vi "RoboDisplay7beingedited.vi"() -> ()   [LabVIEW 2015]
uses:
  GlobalDisplayIndex.vi
  GlobalDataSize.vi
  GlobalInitialParamVals.vi
  GlobalErrorCAN_ID.vi
  ErrorPrevValues.vi
  GlobalErrorCluster.vi
  GlobalLabVIEWStart.vi
  GlobalSpeedUpdateTime.vi
  GlobalPlotUpdateTime.vi
  GlobalSpeedArray.vi
  GlobalDataSelectArray.vi
  GlobalFavoritesList.vi
  GlobalFavorites.vi
  GlobalParamSize.vi
  GlobalFavoriteNames.vi
  GlobalDataFileRefnum7.vi
  GlobalDataPath7.vi
  GlobalRobotOffCheck.vi
  GlobalPrevPage.vi
  GlobalErrorIndex.vi
  GlobalBatteryVoltageID.vi
  GlobalLoadedParams.vi
panel:
  in  "?":T1
  in  "Select":T1
  in  "Select 4":T1
  in  "Select 3":T1
  in  "Load param display file":bool
  out "MCU Elapsed mS 2":u32
  in  "Collect Data":bool
  out "Boolean":bool
  out "graph2labels":string[](array[string])
  out "graph1labels":string[](array[string])
  out "BATTERY VOLTAGE":dbl(knob) scale=20.0..30.0 scale format="%#_3g"
  in  "Tab Control":T2(tab)=enum."Display Data"
  out "Fav Error":bool[](array[boolean])
  in  "Remove":T3
  in  "Fav":T1
  in  "Commit":T4
  out "WAIT":bool
  in  "Reset default":bool
  out "Param #":dbl[](array[numeric])
  in  "Select 2":T5
  in  "Fav Input":dbl[](array[numeric])
  out "Value":dbl[](array[numeric])
  in  "Load":bool
  in  "Save":bool
  out "error":bool[](array[boolean])
  out "Param value":dbl[](array[numeric])
  out "Param #":dbl[](array[numeric])
  out "Param Name":string[](array[string])
  in  "Input":dbl[](array[numeric])
  in  "Page Select":dbl min=0.0 max=50.0 step=1.0
  out "Favorite Parameters":string[](array[string])
  in  "save data":bool
  in  "load data":bool
  out "Value 2":dbl[](array[numeric])
  out "Value 1":dbl[](array[numeric])
  out "Data # 2":dbl[](array[numeric])
  out "Data #":dbl[](array[numeric])
  out "Indicator":bool[](array[boolean])
  out "Array":string[](array[string])
  in  "Page":dbl min=0.0 max=50.0 step=1.0
  out "Number\nSelected":dbl
  out "Indicator 2":bool[](array[boolean])
  out "Array 2":string[](array[string])
  out "Results":T6(array[cluster])
  in  "Search":string
  in  "Search \nButton":bool
  out "# of Results":i32
  in  "Speed Sel 2":enum32{"Slow", "Medium", "Fast"}[](array[radio])
  out "Speed 3":u32[](array[colorbox])
  out "Data Names 2":string[](array[string])
  out "Channel # 2":i16[](array[numeric])
  out "Data Value 2":sgl[](array[numeric]) format="%#_4g"
  out "Speed 2":u32[](array[colorbox])
  out "Data Names 1":string[](array[string])
  out "Channel # 1":i16[](array[numeric])
  out "Data Value 1":sgl[](array[numeric]) format="%#_4g"
  in  "One1":bool[](array[boolean])
  in  "One2":bool[](array[boolean])
  in  "Two1":bool[](array[boolean])
  in  "Two2":bool[](array[boolean])
  in  "Speed Sel":enum32{"Slow", "Medium", "Fast"}[](array[radio])
  in  "Clear Errors":bool
  in  "Pause Button":bool
  out "Error Description":string[](array[string])
  out "Board":string[](array[string])
  out "Error Name":string[](array[string])
  out "Freq.":dbl[](array[numeric])
  out "Time":dbl[](array[numeric])
  out "error message":bool
  out "Board Name 1":string
  out "Graph One":cluster{"Array":u32[], "Array 2":sgl[]}[](graph)
  in  "Graph\non":bool
  out "Error Name 1":string
  out "MCU Elapsed mS":u32 format="%<%H:%M:%S>t"
  in  "stop":bool
  out "Graph Two":cluster{"Array":u32[], "Array 2":sgl[]}[](graph)
  # "Robot Time:"
  # "ms timer:"
  # "DATA COLLECTION"
  # "Board"
  # "OFF"
  # "ON"
  # "Error Name"
  # "RoboDAQ\n\n(Version 7)\n\n\n\n\n\n\nCreated by: John Buzzi, Jason Cortell, Katie Hartl, Carlos Arango\n\nFall 2009"
  # "PLEASE LOOK AT SUGGESTIONS\nTAB IF YOU HAVE HELPFUL \nCOMMENTS!!"
  # "Favorites"
  # "Press [Home] to increment\nPress [End] to decrement"
  # "Press [Page Up] to increment\nPress [Page Down] to decrement"
  # "Select"
  # "Select"
  # "MAX ALLOWED: 48"
  # "NOT WORKING YET\n.\n.\n.\n.\n.\n.\n.\n......................."
  # "CAN ID"
  # "Name"
  # "Search Field"
  # "Note: Add function does not work yet"
  # "# of hits"
  # "Graphs"
  # "Graphs"
  # "Speed\n(S)   (M)   (F)"
  # "Speed\n(S)   (M)   (F)"
  # "Speed"
  # "Speed"
  # "Channel Name"
  # "One"
  # "Two"
  # "Channel Name"
  # "One"
  # "Two"
  # "SUGGESTIONS (double click text box to edit)\n\nMy to do list:\nFix error handling so that it works in the more advanced way that I had intended\nFix bug with speed select when data is de-selected and speeds are incorrect\nradio buttons\nload save data\nadd data by number\nmake index bigger\nslow default speed\n\n\nOther Suggestions/Comments (please add user input so that I can make the program better)\n- (nac) Change default folder for can_id.h and error_id.h to the Ranger Configuration folder\n\n\n\n\nNote: Strikeout = fixed"
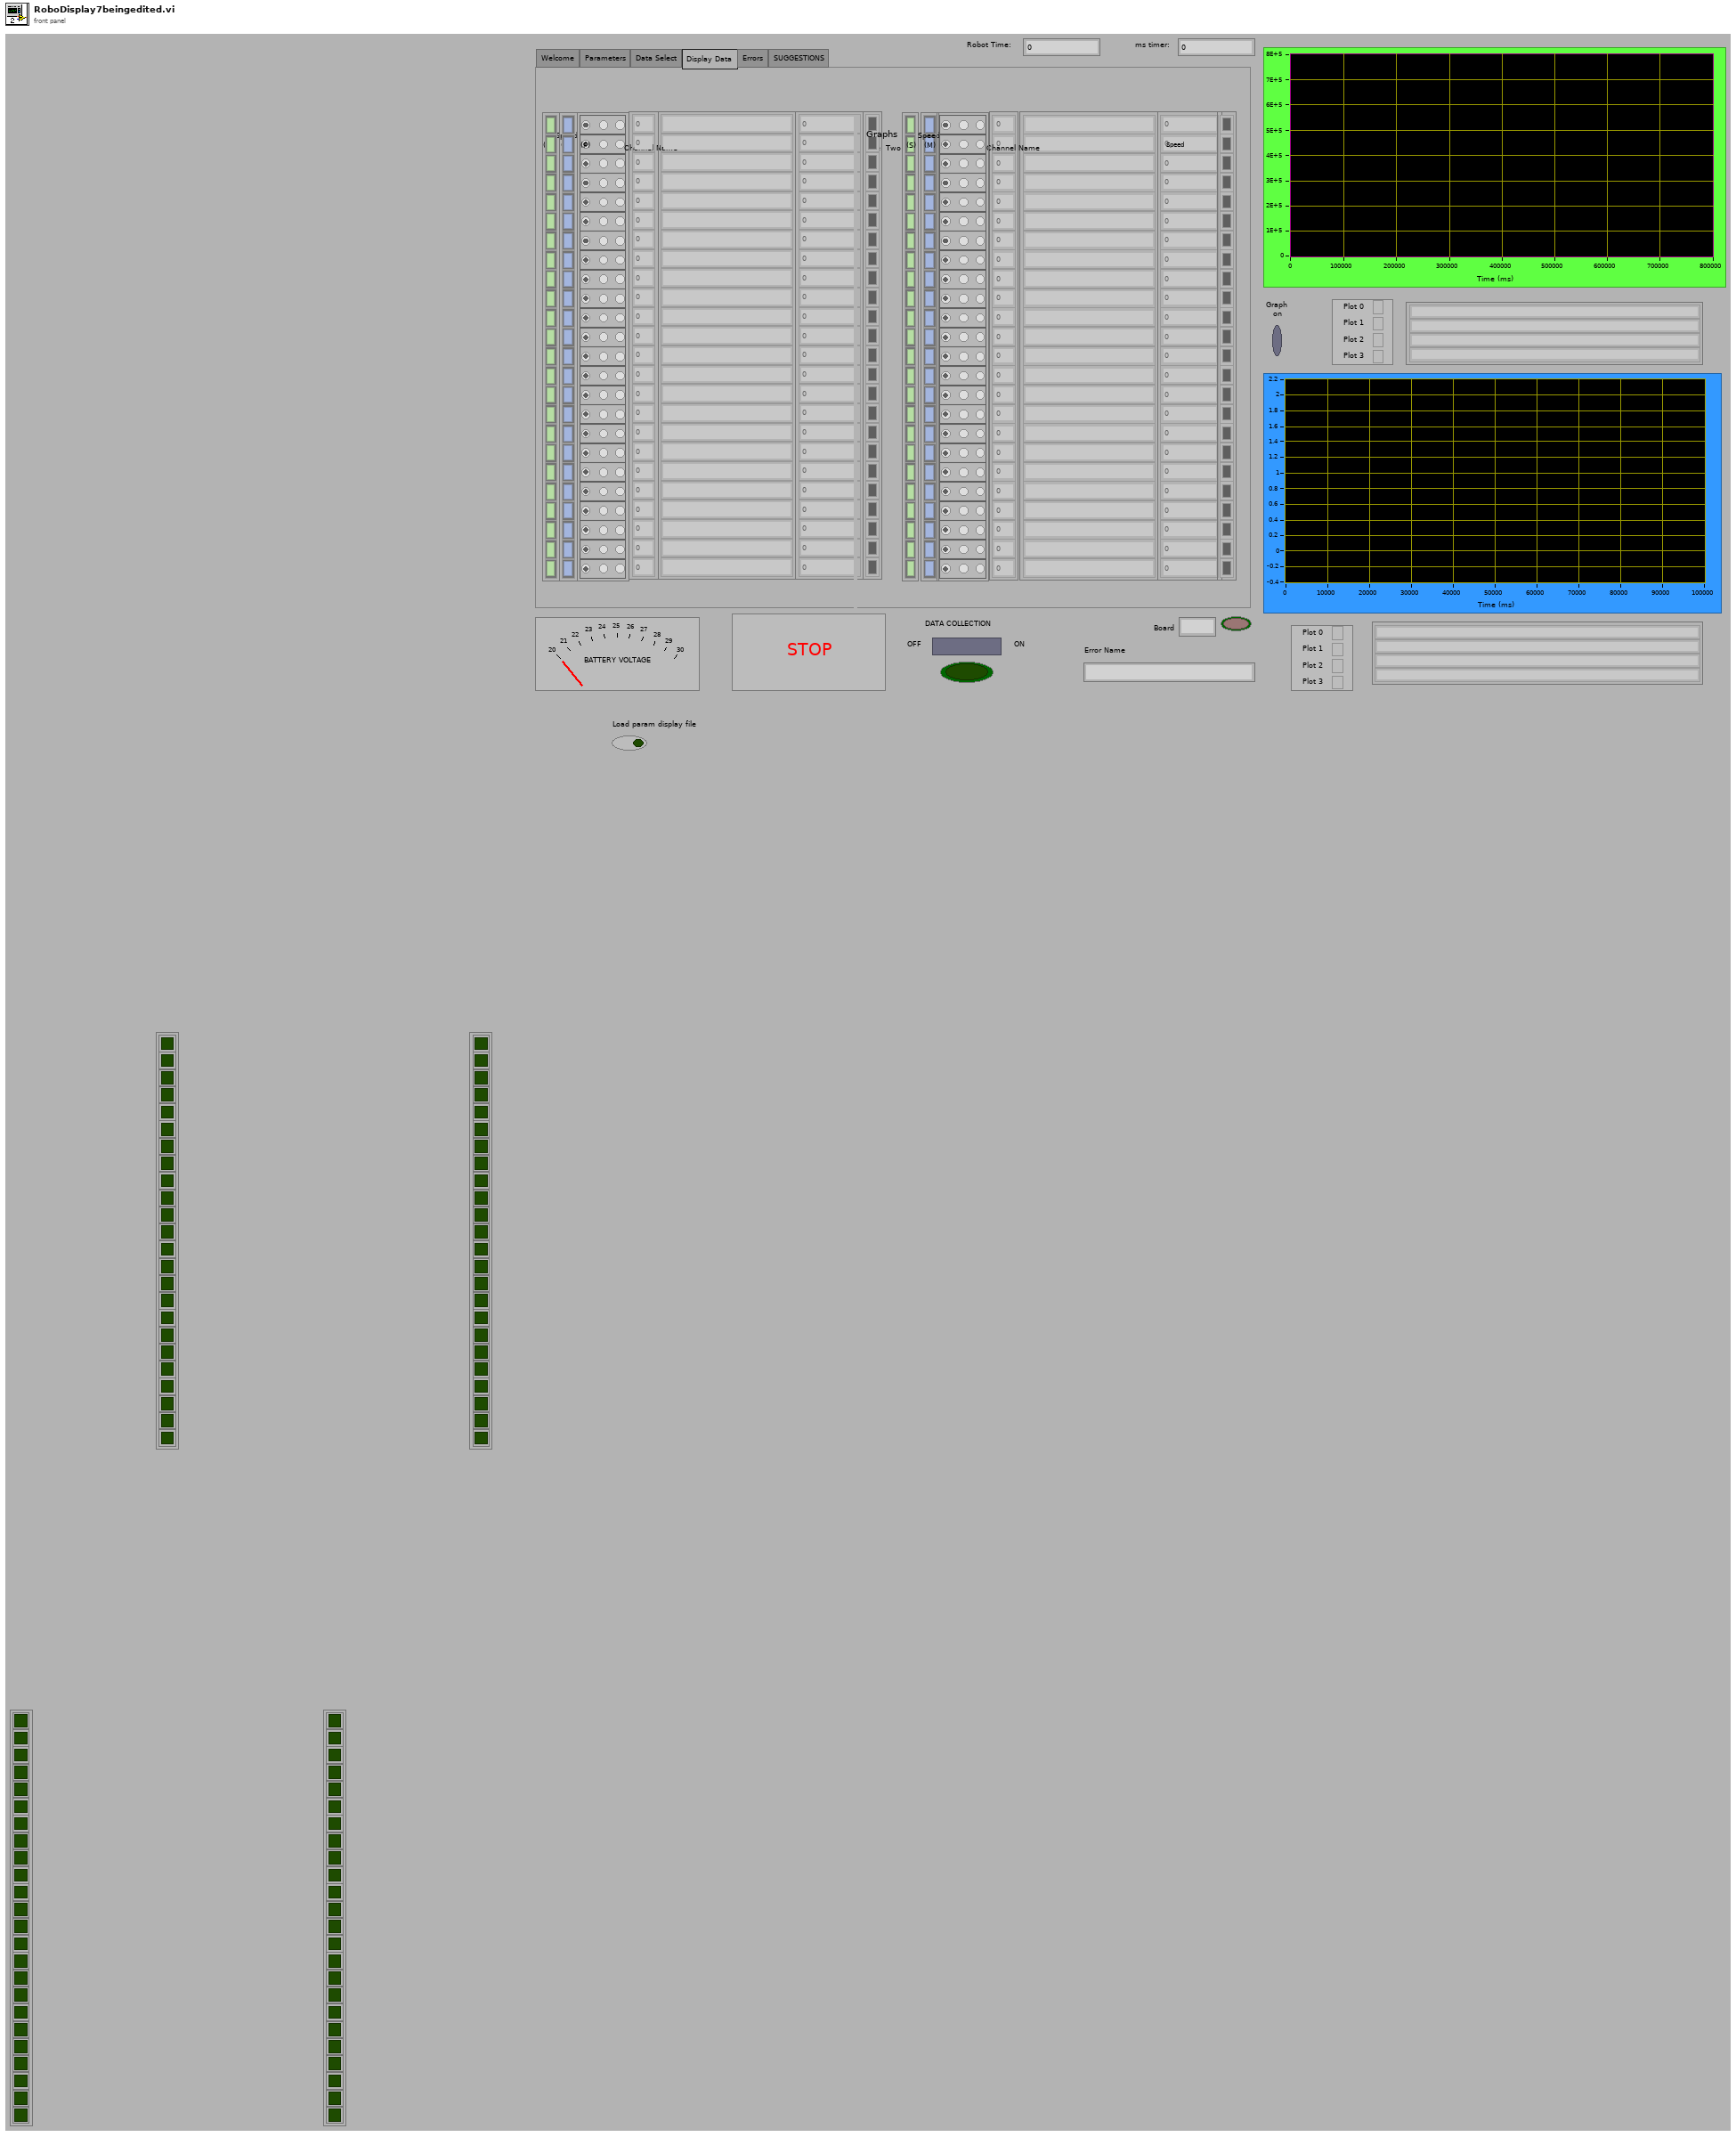
[diagram p1: front panel]
types:
  T1 = cluster{"Boolean 2":bool, "Boolean 3":bool, "Boolean 4":bool, "Boolean 5":bool, "Boolean 6":bool, "Boolean 7":bool, "Boolean 8":bool, "Boolean 9":bool, "Boolean 10":bool, "Boolean 11":bool, "Boolean 12":bool, "Boolean 13":bool, "Boolean 14":bool, "Boolean 15":bool, "Boolean 16":bool, "Boolean 17":bool, "Boolean 18":bool, "Boolean 19":bool, "Boolean 20":bool, "Boolean 21":bool, "Boolean 22":bool, "Boolean 23":bool, "Boolean 24":bool, "Boolean 25":bool}
  T2 = enum32{"Welcome", "Parameters", "Data Select", "Display Data", "Errors", "SUGGESTIONS"}
  T3 = cluster{"X button":bool, "X button 2":bool, "X button 3":bool, "X button 4":bool, "X button 5":bool, "X button 6":bool, "X button 7":bool, "X button 8":bool, "X button 9":bool, "X button 10":bool, "X button 11":bool, "X button 12":bool, "X button 13":bool, "X button 14":bool, "X button 15":bool, "X button 16":bool, "X button 17":bool, "X button 18":bool, "X button 19":bool, "X button 20":bool}
  T4 = cluster{"Boolean":bool, "Boolean 2":bool, "Boolean 3":bool, "Boolean 4":bool, "Boolean 5":bool, "Boolean 6":bool, "Boolean 7":bool, "Boolean 8":bool, "Boolean 9":bool, "Boolean 10":bool, "Boolean 11":bool, "Boolean 12":bool, "Boolean 13":bool, "Boolean 14":bool, "Boolean 15":bool, "Boolean 16":bool, "Boolean 17":bool, "Boolean 18":bool, "Boolean 19":bool, "Boolean 20":bool}
  T5 = cluster{"Boolean":bool, "Boolean 2":bool, "Boolean 3":bool, "Boolean 4":bool, "Boolean 5":bool, "Boolean 6":bool, "Boolean 7":bool, "Boolean 8":bool, "Boolean 9":bool, "Boolean 10":bool, "Boolean 11":bool, "Boolean 12":bool, "Boolean 13":bool, "Boolean 14":bool, "Boolean 15":bool, "Boolean 16":bool, "Boolean 17":bool, "Boolean 18":bool, "Boolean 19":bool, "Boolean 20":bool, "Boolean 21":bool, "Boolean 22":bool, "Boolean 23":bool, "Boolean 24":bool}
  T6 = cluster{"Result Index":dbl, "Results 3":string, "Boolean 2":bool}[]
  T7 = cluster{"Error ID":i32, "Board ID":i32, "Time":u32, "Frequency":i32}[]
  T8 = enum16{"open", "replace", "create", "open or create", "replace or create", "replace or create with confirmation"}
  T9 = cluster{"Numeric":dbl, "String":string, "ignore case? (F)":bool}
  T10 = cluster{"Select 4[0]":bool, "Select 4[1]":bool, "Select 4[2]":bool, "Select 4[3]":bool, "Select 4[4]":bool, "Select 4[5]":bool, "Select 4[6]":bool, "Select 4[7]":bool, "Select 4[8]":bool, "Select 4[9]":bool, "Select 4[10]":bool, "Select 4[11]":bool, "Select 4[12]":bool, "Select 4[13]":bool, "Select 4[14]":bool, "Select 4[15]":bool, "Select 4[16]":bool, "Select 4[17]":bool, "Select 4[18]":bool, "Select 4[19]":bool, "Select 4[20]":bool, "Select 4[21]":bool, "Select 4[22]":bool, "Select 4[23]":bool}
  T11 = cluster{"Select 3[0]":bool, "Select 3[1]":bool, "Select 3[2]":bool, "Select 3[3]":bool, "Select 3[4]":bool, "Select 3[5]":bool, "Select 3[6]":bool, "Select 3[7]":bool, "Select 3[8]":bool, "Select 3[9]":bool, "Select 3[10]":bool, "Select 3[11]":bool, "Select 3[12]":bool, "Select 3[13]":bool, "Select 3[14]":bool, "Select 3[15]":bool, "Select 3[16]":bool, "Select 3[17]":bool, "Select 3[18]":bool, "Select 3[19]":bool, "Select 3[20]":bool, "Select 3[21]":bool, "Select 3[22]":bool, "Select 3[23]":bool}
  T12 = cluster{"Numeric":dbl, "String":string, "ignore case? (F)":bool}[]
  T13 = cluster{"Frequency":dbl, "Description":string, "Error Name":string, "Board Name":string, " Board Source":dbl, "Timestamp":dbl}[]
  T14 = cluster{"Frequency":dbl, "Description":string, "Error Name":string, "Board Name":string, " Board Source":dbl, "Timestamp":dbl}
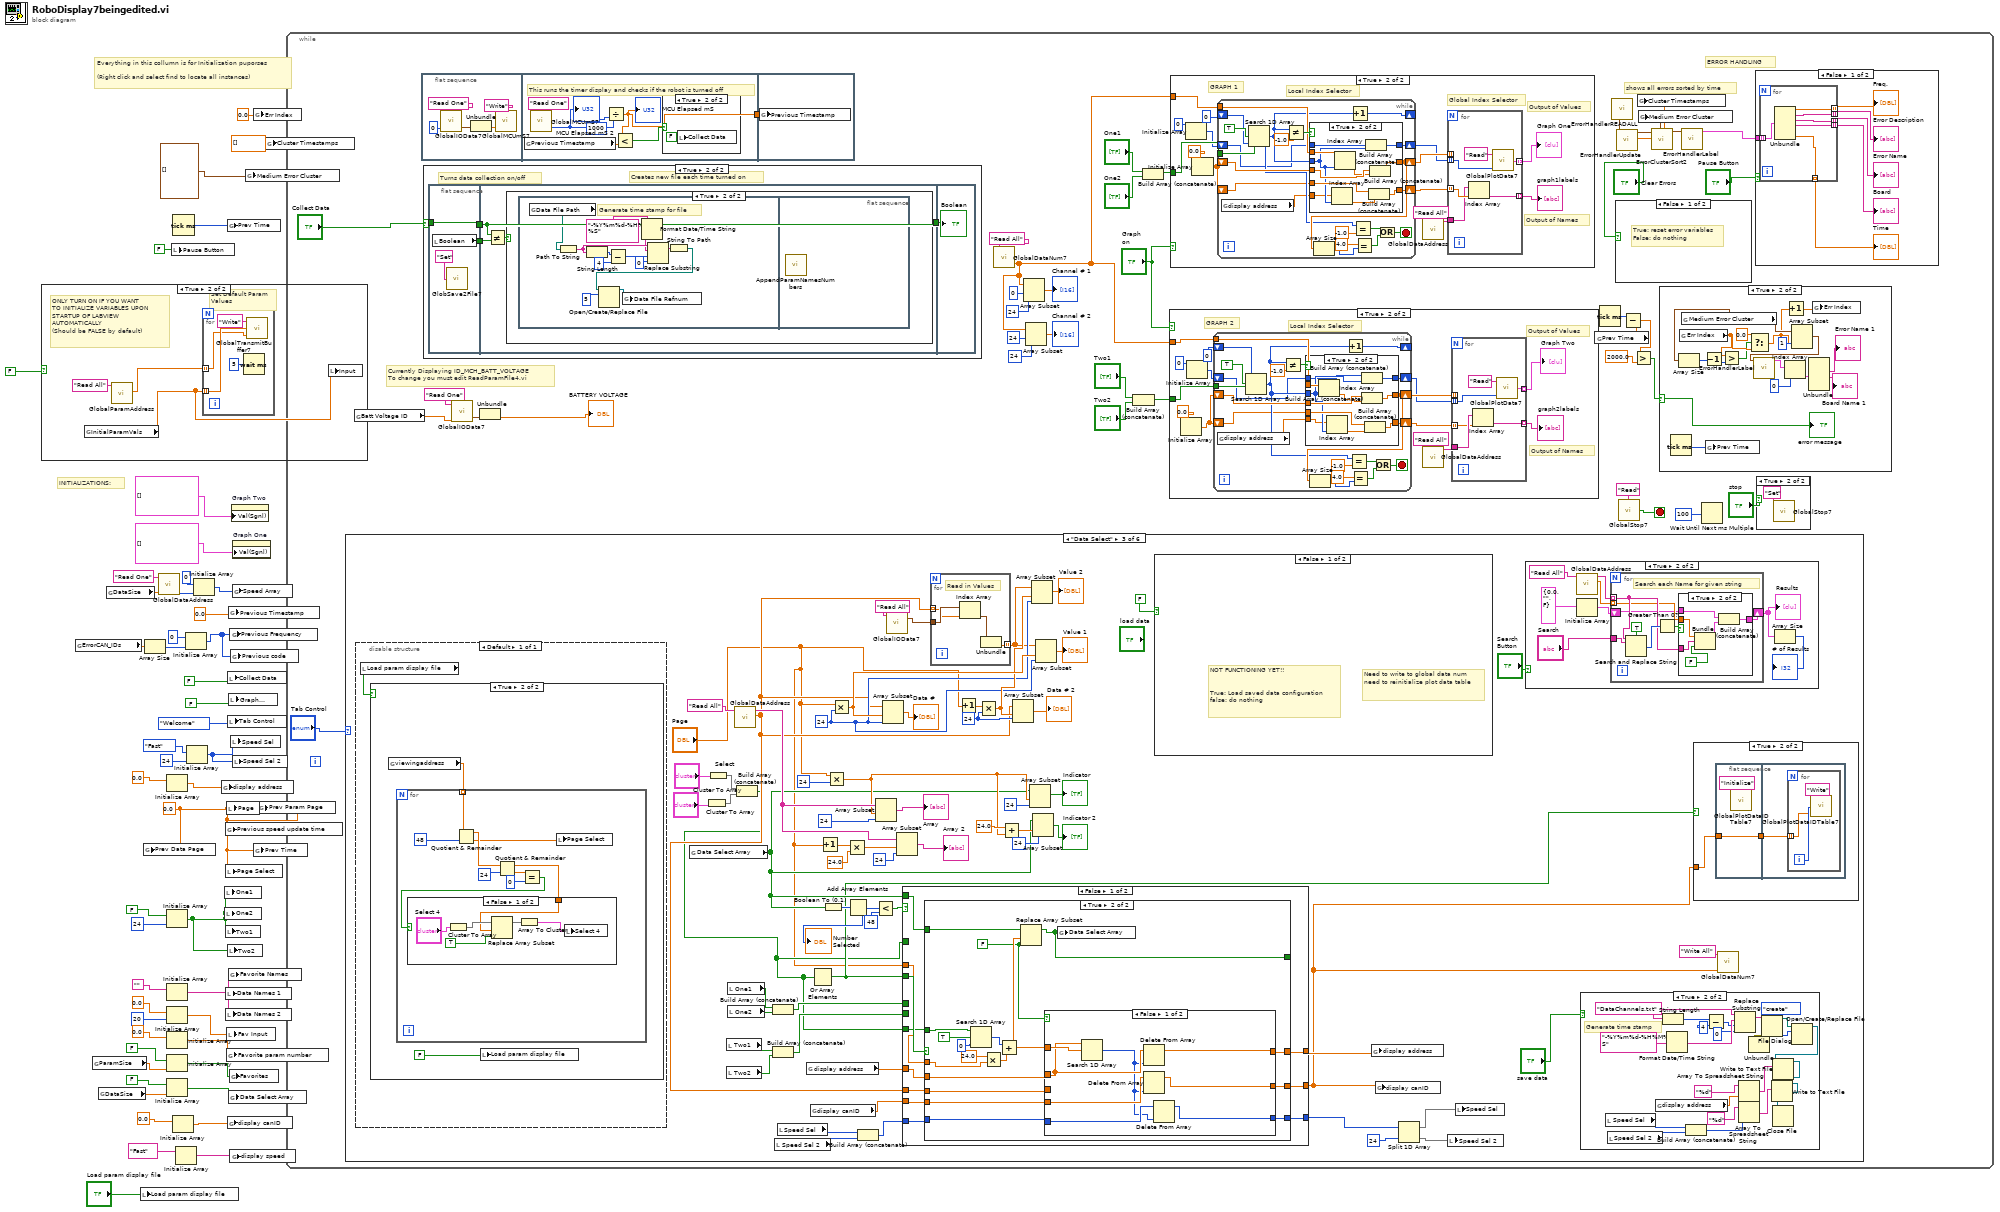
[diagram p0: block diagram]
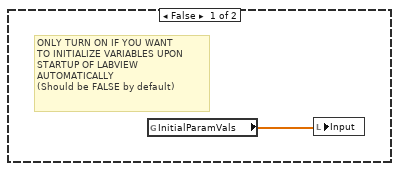
[diagram p2: hidden frame]
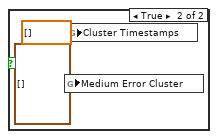
[diagram p3: hidden frame]
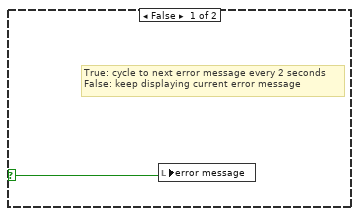
[diagram p4: hidden frame]
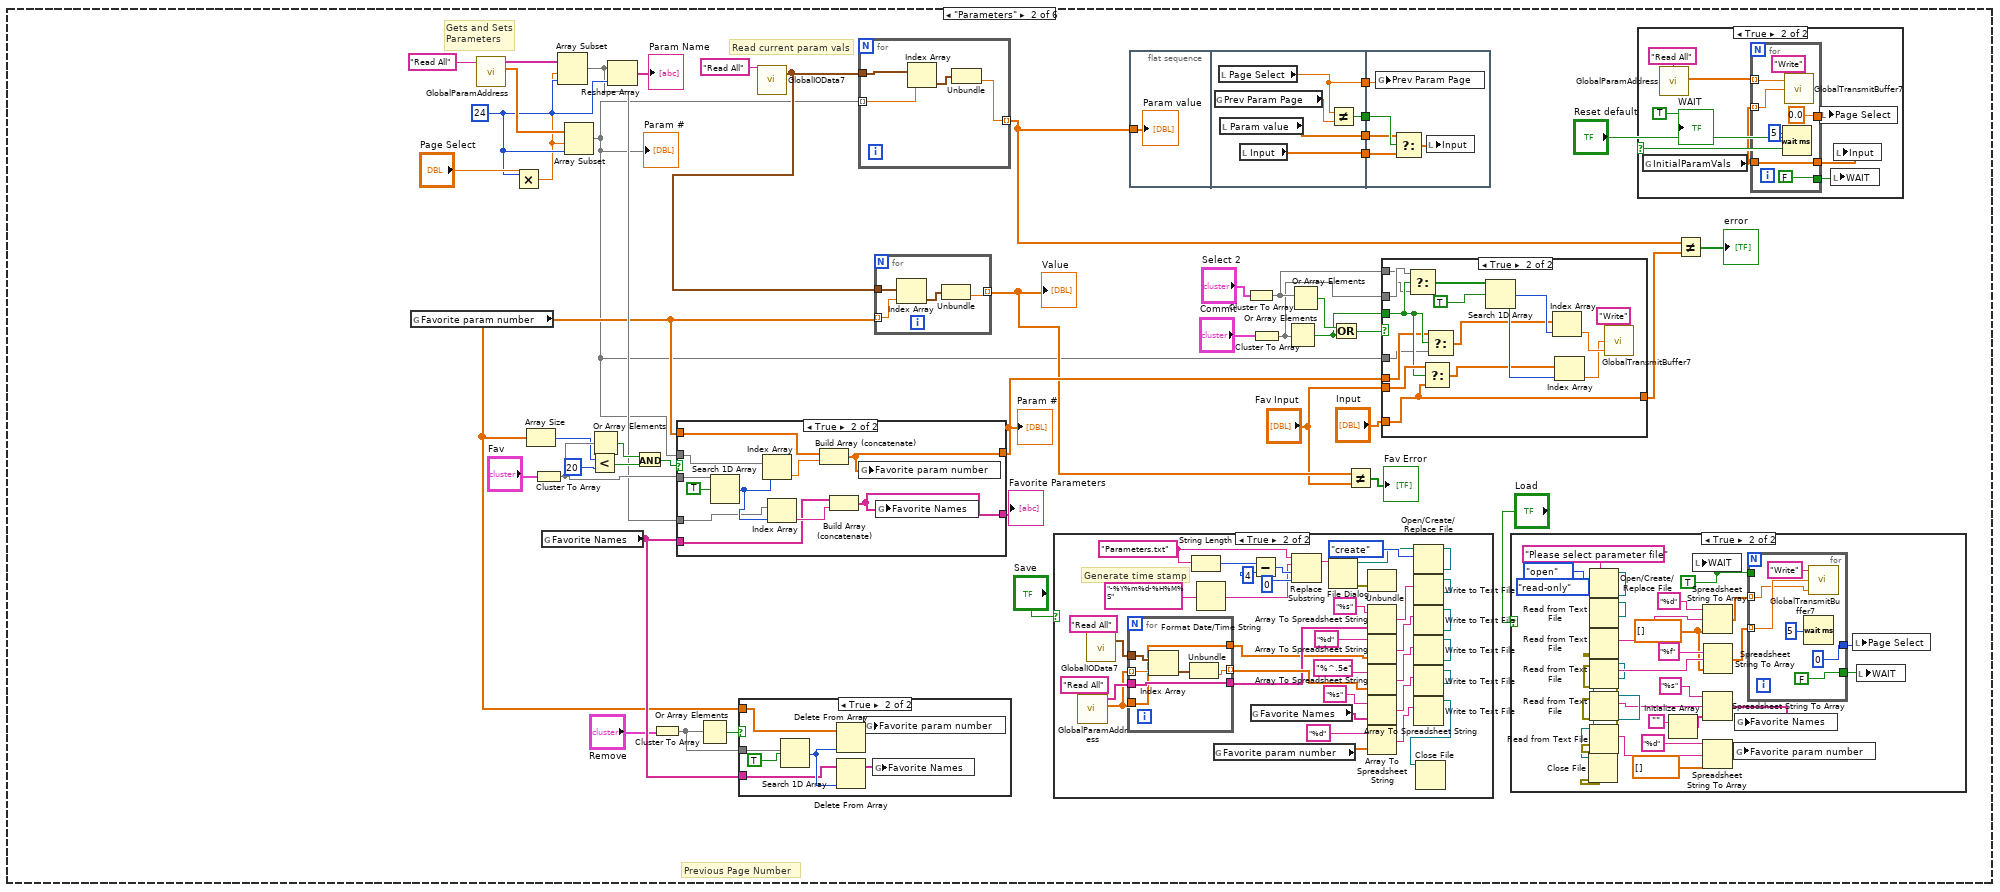
[diagram p12: hidden frame]
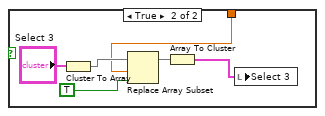
[diagram p20: hidden frame]
diagram:
  w14 = 0.0 ("Previous speed update time")
  # "Everything in this collumn is for Initialization puporses\n\n(Right click and select find to locate all instances)"
  # "INITIALIZATIONS:"
  n1 = case shown="True" FALSE {
    frame False {
      # "ONLY TURN ON IF YOU WANT\nTO INITIALIZE VARIABLES UPON\nSTARTUP OF LABVIEW \nAUTOMATICALLY \n(Should be FALSE by default)"
      n2 = global read "GlobalInitialParamVals.vi" "InitialParamVals"() -> (w49:dbl[])
      n3 = local write "Input"(w49) -> ()
    }
    frame True {
      # "ONLY TURN ON IF YOU WANT\nTO INITIALIZE VARIABLES UPON\nSTARTUP OF LABVIEW \nAUTOMATICALLY \n(Should be FALSE by default)"
      # "Set Default Param\nValues"
      n4 = global read "GlobalInitialParamVals.vi" "InitialParamVals"() -> (w50:dbl[])
      n5 = call "GlobalParamAddress.vi"("Function select"="Read All") -> ("Parameter ID Out"=w52:dbl[])  [unwired: 3 in, 3 out]
      n6 = for {
        tunnel: w52 -> [w54] mode=indexing
        tunnel: w50 -> [w55] mode=indexing
        n7 = Wait (ms)(milliseconds to wait=u32 5) -> ()  [unwired: 1 out]
        n8 = call "GlobalTransmitBuffer7.vi"("Data_ID # in"=w54, "Value in"=w55, "Function select"="Write") -> ()  [unwired: 3 out]
      }
      n9 = local write "Input"(w50) -> ()
    }
  }
  n10 = global read "GlobalErrorCAN_ID.vi" "ErrorCAN_IDs"() -> (w43:dbl[])
  n11 = global read "GlobalParamSize.vi" "ParamSize"() -> (w26:dbl)
  n12 = global read "GlobalDataSize.vi" "DataSize"() -> (w31:dbl)
  n13 = global read "GlobalDataSize.vi" "DataSize"() -> (w35:dbl)
  n14 = local write "Load param display file"("Load param display file") -> ()
  n15 = global write "GlobalPrevPage.vi" "Prev Data Page"(w14) -> ()
  n16 = Array Size(array=w43) -> (size(s)=w41:i32)
  n17 = call "GlobalDataAddress.vi"("Element index"=w35, "Function select"="Read One") -> ("Data ID"=w34:u16)  [unwired: 2 in, 3 out]
  n18 = Initialize Array(0.0 ("Previous speed update time")) -> (w38:dbl[])  [unwired: 1 in]
  n19 = Initialize Array(FALSE ("Graph\non"), 24 ("dimension size")) -> (w24:bool[])
  n20 = Initialize Array("") -> (w20:string[])  [unwired: 1 in]
  n21 = Initialize Array(0.0 ("Previous speed update time"), 20 ("dimension size")) -> (w22:dbl[])
  n22 = Initialize Array(0.0 ("Previous speed update time")) -> (w28:dbl[])  [unwired: 1 in]
  n23 = Initialize Array(FALSE, w26) -> (w25:bool[])
  n24 = Initialize Array(FALSE, w31) -> (w29:bool[])
  n25 = local write "Pause Button"(FALSE ("Pause Button")) -> ()
  n26 = Initialize Array(0.0 ("Previous speed update time")) -> (w12:dbl[])  [unwired: 1 in]
  n27 = Tick Count (ms)() -> (millisecond timer value=w3:u32)
  n28 = Initialize Array("Fast" ("Combo Box")) -> (w10:string[])  [unwired: 1 in]
  n29 = Initialize Array(0 ("dimension size"), w41) -> (w40:i32[])
  n30 = Initialize Array(enum32{"Slow", "Medium", "Fast"}."Fast" ("Radio Buttons 2"), 24 ("dimension size")) -> (w4:enum32{"Slow", "Medium", "Fast"}[])
  n31 = Initialize Array(0, w34) -> (w32:i32[])
  n32 = global write "GlobalDisplayIndex.vi" "display address"(w38) -> ()
  n33 = local write "One1"(w24) -> ()
  n34 = local write "One2"(w24) -> ()
  n35 = local write "Two1"(w24) -> ()
  n36 = global write "GlobalSpeedUpdateTime.vi" "Previous speed update time"(w14) -> ()
  n37 = local write "Page Select"(w14) -> ()
  n38 = local write "Data Names 1"(w20) -> ()
  n39 = local write "Data Names 2"(w20) -> ()
  n40 = local write "Page"(w14) -> ()
  n41 = local write "Fav Input"(w22) -> ()
  n42 = global write "GlobalFavoritesList.vi" "Favorite param number"(w28) -> ()
  n43 = global write "GlobalPlotUpdateTime.vi" "Prev Time"(w3) -> ()
  n44 = local write "Two2"(w24) -> ()
  n45 = global write "GlobalDisplayIndex.vi" "display canID"(w12) -> ()
  n46 = local write "Collect Data"(FALSE ("Boolean 2")) -> ()
  n47 = local write "Tab Control"(T2."Welcome" ("Tab Control")) -> ()
  n48 = global write "GlobalRobotOffCheck.vi" "Previous Timestamp"(0.0 ("Previous Timestamp")) -> ()
  n49 = local write "Graph\non"(FALSE ("Graph\non")) -> ()
  n50 = global write "GlobalFavoriteNames.vi" "Favorite Names"(w20) -> ()
  n51 = global write "GlobalDataSelectArray.vi" "Data Select Array"(w29) -> ()
  n52 = global write "GlobalFavorites.vi" "Favorites"(w25) -> ()
  n53 = global write "ErrorPrevValues.vi" "Previous Frequency"(w40) -> ()
  n54 = global write "GlobalDisplayIndex.vi" "display speed"(w10) -> ()
  n55 = global write "ErrorPrevValues.vi" "Previous code"(w40) -> ()
  n56 = local write "Speed Sel"(w4) -> ()
  n57 = property on="Graph Two" class="XYGraph (strict)"("Val(Sgnl)"=cluster{"Array":dbl[], "Array 2":dbl[]}[] [] ("Value (Signaling)")) -> ()  [unwired: 2 in, 2 out]
  n58 = global write "GlobalSpeedArray.vi" "Speed Array"(w32) -> ()
  n59 = local write "Speed Sel 2"(w4) -> ()
  n60 = property on="Graph One" class="XYGraph (strict)"("Val(Sgnl)"=cluster{"Array":dbl[], "Array 2":dbl[]}[] [] ("Value (Signaling)")) -> ()  [unwired: 2 in, 2 out]
  n61 = global write "GlobalErrorCluster.vi" "Medium Error Cluster"(T7 [] ("Medium Error Cluster")) -> ()
  n62 = global write "GlobalErrorIndex.vi" "Err Index"(0.0 ("Err Index")) -> ()
  n63 = global write "GlobalPlotUpdateTime.vi" "Prev Time"(w14) -> ()
  n64 = global write "GlobalPrevPage.vi" "Prev Param Page"(w14) -> ()
  n65 = global write "GlobalErrorCluster.vi" "Cluster Timestamps"(dbl[] [] ("Cluster Timestamps")) -> ()
  n66 = while {
    stop <- w92 stop-if-true
    # "shows all errors sorted by time"
    # "Currently Displaying ID_MCH_BATT_VOLTAGE\nTo change you must edit ReadParamFile4.vi"
    # "ERROR HANDLING"
    n67 = case shown="\"Data Select\"" "Tab Control" {
      frame "Welcome", Default {
        # "Introduction Page"
      }
      frame "Parameters" {
        w278 = 24 ("index")
        # "Read current param vals"
        # "Previous Page Number"
        # "Gets and Sets\nParameters"
        n68 = global read "GlobalFavoritesList.vi" "Favorite param number"() -> (w263:dbl[])
        n69 = call "GlobalParamAddress.vi"("Function select"="Read All") -> ("Parameter ID Out"=w291:dbl[], "Parameter Names Out"=w290:string[])  [unwired: 3 in, 2 out]
        n70 = Multiply(x=w278, y="Page Select") -> (x*y=w277:dbl)
        n71 = Array Size(array=w263) -> (size(s)=w274:i32)
        n72 = Cluster To Array(cluster="Fav") -> (array=w275:bool[])
        n73 = global read "GlobalFavoriteNames.vi" "Favorite Names"() -> (w264:string[])
        n74 = Array Subset(array=w290, index=w277, length=w278) -> (w267:string[])
        n75 = Array Subset(array=w291, index=w277, length=w278) -> (w251:dbl[])
        "Param #" <- w251
        n76 = Less?(x=w274, y=20) -> (x < y?=w270:bool)
        n77 = Or Array Elements(Boolean array=w275) -> (logical OR=w271:bool)
        n78 = Reshape Array(w267, w278) -> (→"Param Name":string[])
        n79 = And(x=w271, y=w270) -> (x .and. y?=w272:bool)
        n80 = Cluster To Array(cluster="Remove") -> (array=w261:bool[])
        n81 = case shown="True" w272 {
          tunnel: w251 -> [_ w331]
          tunnel: w275 -> [_ w329]
          tunnel: w263 -> [w320 w327]
          tunnel: [w320 w326] -> w269
          tunnel: w264 -> [w319 w324]
          tunnel: w267 -> [_ w322]
          tunnel: [w319 w321] -> w266
          frame False {
            # "True: Add a favorite\nFalse: Do nothing"
          }
          frame True {
            n82 = Search 1D Array(1D array=w329, element=TRUE) -> (index of element=w323:i32)  [unwired: 1 in]
            n83 = Index Array(array=w331, index=w323) -> (element=w330:dbl)
            n84 = Index Array(array=w322, index=w323) -> (element=w325:string)
            n85 = Build Array (concatenate)(w327, w330) -> (w326:dbl[])
            n86 = Build Array (concatenate)(w324, w325) -> (w321:string[])
            n87 = global write "GlobalFavoritesList.vi" "Favorite param number"(w326) -> ()
            n88 = global write "GlobalFavoriteNames.vi" "Favorite Names"(w321) -> ()
          }
        }
        "Param #" <- w269
        "Favorite Parameters" <- w266
        n89 = Or Array Elements(Boolean array=w261) -> (logical OR=w265:bool)
        n90 = case shown="True" w265 {
          tunnel: w261 -> [_ w313]
          tunnel: w264 -> [_ w309]
          tunnel: w263 -> [_ w311]
          frame False {
            # "True: Remove a favorite\nFalse: do nothing"
          }
          frame True {
            n91 = Search 1D Array(1D array=w313, element=TRUE) -> (index of element=w312:i32)  [unwired: 1 in]
            n92 = Delete From Array(array=w311, index=w312) -> (array with subset deleted=w310:dbl[])  [unwired: 1 in, 1 out]
            n93 = Delete From Array(array=w309, index=w312) -> (array with subset deleted=w308:string[])  [unwired: 1 in, 1 out]
            n94 = global write "GlobalFavoritesList.vi" "Favorite param number"(w310) -> ()
            n95 = global write "GlobalFavoriteNames.vi" "Favorite Names"(w308) -> ()
          }
        }
        n96 = call "GlobalIOData7.vi"("Function select"="Read All") -> ("Array"=w268:cluster{"Time":u32, "Value":sgl}[])  [unwired: 4 in, 1 out]
        n97 = for {
          tunnel: w251 -> [w393] mode=indexing
          tunnel: w268 -> [w392]
          tunnel: [w390] -> w252 mode=indexing
          n98 = Index Array(array=w392, index=w393) -> (element=w391:cluster{"Time":u32, "Value":sgl})
          n99 = Unbundle(w391) -> ("Value"=w390:sgl)  [unwired: 1 out]
        }
        n100 = for {
          tunnel: w263 -> [w318] mode=indexing
          tunnel: w268 -> [w317]
          tunnel: [w315] -> w260 mode=indexing
          n101 = Index Array(array=w317, index=w318) -> (element=w316:cluster{"Time":u32, "Value":sgl})
          n102 = Unbundle(w316) -> ("Value"=w315:sgl)  [unwired: 1 out]
        }
        "Value" <- w260
        n103 = case shown="True" "Save" {
          frame False {
            # "True: Save parameters and favorites\nFalse: do nothing"
          }
          frame True {
            w353 = "Parameters.txt" ("Default file name")
            # "Generate time stamp"
            n104 = call "GlobalParamAddress.vi"("Function select"="Read All") -> ("Parameter ID Out"=w348:dbl[], "Parameter Names Out"=w367:string[])  [unwired: 3 in, 2 out]
            n105 = call "GlobalIOData7.vi"("Function select"="Read All") -> ("Array"=w365:cluster{"Time":u32, "Value":sgl}[])  [unwired: 4 in, 1 out]
            n106 = for {
              tunnel: w367 -> [w371]
              tunnel: w348 -> [w375] mode=indexing
              tunnel: w365 -> [w374]
              tunnel: [w372] -> w364 mode=indexing
              tunnel: [w371] -> w362
              tunnel: w348 -> [w370]
              tunnel: [w370] -> w343
              n107 = Index Array(array=w374, index=w375) -> (element=w373:cluster{"Time":u32, "Value":sgl})
              n108 = Unbundle(w373) -> ("Value"=w372:sgl)  [unwired: 1 out]
            }
            n109 = String Length(string=w353) -> (length=w355:i32)
            n110 = Format Date/Time String(time format string (%c)="-%Y%m%d-%H%M%S") -> (date/time string=w349:string)  [unwired: 2 in]
            n111 = global read "GlobalFavoritesList.vi" "Favorite param number"() -> (w336:dbl[])
            n112 = global read "GlobalFavoriteNames.vi" "Favorite Names"() -> (w337:string[])
            n113 = Subtract(x=w355, y=4) -> (x-y=w351:i32)
            n114 = Replace Substring(2:0, 3:w351, 4:w349, 5:w353) -> (1:w354:string)  [unwired: 1 out]
            n115 = File Dialog(9:w354) -> (0:w357:errorcluster, 3:w356:path)  [unwired: 6 in, 2 out]
            n116 = Unbundle(w357) -> ()  [unwired: 3 out]
            n117 = Array To Spreadsheet String(array=w362, 3:"%s") -> (spreadsheet string=w359:string)  [unwired: 1 in]
            n118 = Array To Spreadsheet String(array=w343, 3:"%d") -> (spreadsheet string=w344:string)  [unwired: 1 in]
            n119 = Array To Spreadsheet String(array=w364, 3:"%^.5e") -> (spreadsheet string=w342:string)  [unwired: 1 in]
            n120 = Array To Spreadsheet String(array=w337, 3:"%s") -> (spreadsheet string=w339:string)  [unwired: 1 in]
            n121 = Array To Spreadsheet String(array=w336, 3:"%d") -> (spreadsheet string=w338:string)  [unwired: 1 in]
            n122 = Open/Create/Replace File(file path (use dialog)=w356, operation (0:open)=T8."create") -> (refnum out=w358:refnum<file>, error out=w333:errorcluster)  [unwired: 4 in, 1 out]
            n123 = Write to Text File(file (use dialog)=w358, text=w359, error in=w333) -> (refnum out=w347:refnum<file>)  [unwired: 1 in, 2 out]
            n124 = Write to Text File(file (use dialog)=w347, text=w344) -> (refnum out=w346:refnum<file>)  [unwired: 2 in, 2 out]
            n125 = Write to Text File(file (use dialog)=w346, text=w342) -> (refnum out=w341:refnum<file>)  [unwired: 2 in, 2 out]
            n126 = Write to Text File(file (use dialog)=w341, text=w339) -> (refnum out=w340:refnum<file>)  [unwired: 2 in, 2 out]
            n127 = Write to Text File(file (use dialog)=w340, text=w338) -> (refnum out=w332:refnum<file>)  [unwired: 2 in, 2 out]
            n128 = Close File(refnum=w332) -> ()  [unwired: 1 in, 2 out]
          }
        }
        n129 = flat-sequence {
          tunnel: w252 -> [w297]
          tunnel: [w301] -> w257
          tunnel: [w300] -> w256
          tunnel: [w299] -> w254
          tunnel: [w298] -> w253
          tunnel: w257 -> [w307]
          tunnel: w256 -> [w305]
          tunnel: w253 -> [w304]
          tunnel: w254 -> [w303]
          frame #0 {
            "Param value" <- w297
          }
          frame #1 {
            n130 = global read "GlobalPrevPage.vi" "Prev Param Page"() -> (w302:dbl)
            n131 = local read "Page Select"() -> (w301:dbl)
            n132 = local read "Param value"() -> (w298:dbl[])
            n133 = local read "Input"() -> (w299:dbl[])
            n134 = Not Equal?(x=w301, y=w302) -> (x != y?=w300:bool)
          }
          frame #2 {
            n135 = global write "GlobalPrevPage.vi" "Prev Param Page"(w307) -> ()
            n136 = Select(t=w304, s=w305, f=w303) -> (s? t:f=w306:dbl[])
            n137 = local write "Input"(w306) -> ()
          }
        }
        n138 = Cluster To Array(cluster="Select 2") -> (array=w286:bool[])
        n139 = Cluster To Array(cluster="Commit") -> (array=w279:bool[])
        n140 = Or Array Elements(Boolean array=w279) -> (logical OR=w280:bool)
        n141 = Or Array Elements(Boolean array=w286) -> (logical OR=w282:bool)
        n142 = Or(x=w282, y=w280) -> (x .or. y?=w281:bool)
        n143 = Not Equal?(x=w260, y="Fav Input") -> (x != y?=→"Fav Error":bool[])
        n144 = case shown="True" w281 {
          tunnel: w286 -> [_ w395]
          tunnel: "Input" -> [w394 w403]
          tunnel: [w394 w403] -> w293
          tunnel: w251 -> [_ w397]
          tunnel: w280 -> [_ w400]
          tunnel: "Fav Input" -> [_ w402]
          tunnel: w279 -> [_ w396]
          tunnel: w269 -> [_ w398]
          frame False {
            # "True: commit selected parameter value to the\ntransmit buffer \n\nFalse: do nothing"
          }
          frame True {
            n145 = Select(t=w396, s=w400, f=w395) -> (s? t:f=w401:bool[])
            n146 = Select(t=w402, s=w400, f=w403) -> (s? t:f=w404:dbl[])
            n147 = Select(t=w398, s=w400, f=w397) -> (s? t:f=w399:dbl[])
            n148 = Search 1D Array(1D array=w401, element=TRUE) -> (index of element=w408:i32)  [unwired: 1 in]
            n149 = Index Array(array=w399, index=w408) -> (element=w407:dbl)
            n150 = Index Array(array=w404, index=w408) -> (element=w406:dbl)
            n151 = call "GlobalTransmitBuffer7.vi"("Data_ID # in"=w407, "Value in"=w406, "Function select"="Write") -> ()  [unwired: 3 out]
          }
        }
        n152 = case shown="True" "Load" {
          frame False {
            # "True: Load saved parameters and favorites\nFalse: Do nothing"
          }
          frame True {
            w429 = sgl[] []
            w427 = TRUE ("Wait")
            n153 = Open/Create/Replace File(prompt="Please select parameter file", operation (0:open)=T8."open", access (0:read/write)=enum16{"read/write", "read-only", "write-only"}."read-only") -> (refnum out=w440:refnum<file>)  [unwired: 3 in, 2 out]
            n154 = Read from Text File(file (use dialog)=w440) -> (refnum out=w438:refnum<file>, error out=w439:errorcluster)  [unwired: 3 in, 2 out]
            n155 = Read from Text File(file (use dialog)=w438, error in=w439) -> (refnum out=w436:refnum<file>, text=w435:string, error out=w437:errorcluster)  [unwired: 2 in, 1 out]
            n156 = Read from Text File(file (use dialog)=w436, error in=w437) -> (refnum out=w423:refnum<file>, text=w433:string, error out=w424:errorcluster)  [unwired: 2 in, 1 out]
            n157 = Read from Text File(file (use dialog)=w423, error in=w424) -> (refnum out=w421:refnum<file>, text=w420:string, error out=w422:errorcluster)  [unwired: 2 in, 1 out]
            n158 = Read from Text File(file (use dialog)=w421, error in=w422) -> (refnum out=w410:refnum<file>, text=w417:string, error out=w411:errorcluster)  [unwired: 2 in, 1 out]
            n159 = Close File(refnum=w410, error in=w411) -> ()  [unwired: 2 out]
            n160 = Initialize Array("") -> (w414:string[])  [unwired: 1 in]
            n161 = local write "WAIT"(w427) -> ()
            n162 = Spreadsheet String To Array(format string="%d", spreadsheet string=w435, array type (2D Dbl)=w429) -> (array=w434:sgl[])  [unwired: 1 in]
            n163 = Spreadsheet String To Array(format string="%s", spreadsheet string=w420, array type (2D Dbl)=w414) -> (array=w413:string[])  [unwired: 1 in]
            n164 = Spreadsheet String To Array(format string="%d", spreadsheet string=w417, array type (2D Dbl)=sgl[] []) -> (array=w418:sgl[])  [unwired: 1 in]
            n165 = Spreadsheet String To Array(format string="%f", spreadsheet string=w433, array type (2D Dbl)=w429) -> (array=w430:sgl[])  [unwired: 1 in]
            n166 = global write "GlobalFavoritesList.vi" "Favorite param number"(w418) -> ()
            n167 = global write "GlobalFavoriteNames.vi" "Favorite Names"(w413) -> ()
            n168 = for {
              tunnel: w434 -> [w446] mode=indexing
              tunnel: w430 -> [w447] mode=indexing
              tunnel: [FALSE ("Wait")] -> w442
              tunnel: [0] -> w428
              tunnel: w427 -> [_]
              n169 = Wait (ms)(milliseconds to wait=u32 5) -> ()  [unwired: 1 out]
              n170 = call "GlobalTransmitBuffer7.vi"("Data_ID # in"=w446, "Value in"=w447, "Function select"="Write") -> ()  [unwired: 3 out]
            }
            n171 = local write "Page Select"(w428) -> ()
            n172 = local write "WAIT"(w442) -> ()
          }
        }
        n173 = case shown="True" "Reset default" {
          frame False {
            # "True: Reset to default parameters\nFalse: Do nothing"
          }
          frame True {
            n174 = global read "GlobalInitialParamVals.vi" "InitialParamVals"() -> (w378:dbl[])
            n175 = call "GlobalParamAddress.vi"("Function select"="Read All") -> ("Parameter ID Out"=w381:dbl[])  [unwired: 3 in, 3 out]
            n176 = for {
              tunnel: w381 -> [w387] mode=indexing
              tunnel: w378 -> [w388] mode=indexing
              tunnel: [FALSE ("Wait")] -> w380
              tunnel: [w384] -> w377
              tunnel: w378 -> [w384]
              tunnel: [0.0 ("Page Select")] -> w376
              n177 = Wait (ms)(milliseconds to wait=u32 5) -> ()  [unwired: 1 out]
              n178 = call "GlobalTransmitBuffer7.vi"("Data_ID # in"=w387, "Value in"=w388, "Function select"="Write") -> ()  [unwired: 3 out]
            }
            n179 = local write "Page Select"(w376) -> ()
            n180 = local write "WAIT"(w380) -> ()
            n181 = local write "Input"(w377) -> ()
            "WAIT" <- TRUE ("Wait")
          }
        }
        n182 = Not Equal?(x=w252, y=w293) -> (x != y?=→"error":bool[])
      }
      frame "Data Select" {
        w490 = 24 ("length")
        w481 = 24 ("length")
        n183 = disable-structure shown="Default" {
          frame Enabled {
            n184 = local read "Load param display file"() -> (w512:bool)
            n185 = case shown="True" w512 {
              frame False {
              }
              frame True {
                n186 = global read "GlobalLoadedParams.vi" "viewingaddress"() -> (w513:dbl[])
                n187 = for {
                  tunnel: w513 -> [w523] mode=indexing
                  n188 = Quotient & Remainder(x=w523, y=i16 48) -> (x-y*floor(x/y)=w521:dbl, floor(x/y)=w515:dbl)
                  n189 = Quotient & Remainder(x=w521, y=i16 24) -> (x-y*floor(x/y)=w516:dbl, floor(x/y)=w519:dbl)
                  n190 = Equal?(x=w519, y=i16 0) -> (x = y?=w518:bool)
                  n191 = case shown="False" w518 {
                    tunnel: w516 -> [w524 w530]
                    frame False {
                      n192 = Cluster To Array(cluster="Select 4") -> (array=w528:bool[])
                      n193 = Replace Array Subset(array=w528, new element=TRUE, index=w524) -> (w527:bool[])
                      n194 = Array To Cluster(array=w527) -> (cluster=w526:T10)
                      n195 = local write "Select 4"(w526) -> ()
                    }
                    frame True {
                      n196 = Cluster To Array(cluster="Select 3") -> (array=w533:bool[])
                      n197 = Replace Array Subset(array=w533, new element=TRUE, index=w530) -> (w534:bool[])
                      n198 = Array To Cluster(array=w534) -> (cluster=w535:T11)
                      n199 = local write "Select 3"(w535) -> ()
                    }
                  }
                  n200 = local write "Page Select"(w515) -> ()
                }
                n201 = local write "Load param display file"(FALSE) -> ()
              }
            }
          }
        }
        n202 = global read "GlobalDataSelectArray.vi" "Data Select Array"() -> (w477:bool[])
        n203 = Cluster To Array(cluster="?") -> (array=w454:bool[])
        n204 = Cluster To Array(cluster="Select") -> (array=w452:bool[])
        n205 = local read "Two1"() -> (w466:bool[])
        n206 = local read "Two2"() -> (w467:bool[])
        n207 = local read "One1"() -> (w464:bool[])
        n208 = local read "One2"() -> (w465:bool[])
        n209 = call "GlobalDataAddress.vi"("Function select"="Read All") -> ("Data ID Out"=w476:dbl[], "Data Names Out"=w496:string[])  [unwired: 3 in, 2 out]
        n210 = Build Array (concatenate)(w452, w454) -> (w450:bool[])
        n211 = Build Array (concatenate)(w464, w465) -> (w462:bool[])
        n212 = Build Array (concatenate)(w466, w467) -> (w463:bool[])
        n213 = local read "Speed Sel 2"() -> (w459:enum32{"Slow", "Medium", "Fast"}[])
        n214 = local read "Speed Sel"() -> (w458:enum32{"Slow", "Medium", "Fast"}[])
        n215 = global read "GlobalDisplayIndex.vi" "display address"() -> (w475:dbl[])
        n216 = global read "GlobalDisplayIndex.vi" "display canID"() -> (w474:dbl[])
        n217 = Or Array Elements(Boolean array=w450) -> (logical OR=w468:bool)
        n218 = Increment(x="Page") -> (x+1=w491:dbl)
        n219 = Boolean To (0,1)(Boolean=w477) -> (0, 1=w508:i16[])
        n220 = Multiply(x="Page", y=24 ("length")) -> (x*y=w494:dbl)
        n221 = Multiply(x="Page", y=w481) -> (x*y=w483:dbl)
        n222 = Multiply(x=w491, y=24.0) -> (x*y=w493:dbl)
        n223 = Add Array Elements(numeric array=w508) -> (sum=w486:i16)
        "Number\nSelected" <- w486
        n224 = Build Array (concatenate)(w458, w459) -> (w471:enum32{"Slow", "Medium", "Fast"}[])
        n225 = Array Subset(array=w496, index=w494, length=24) -> (→"Array":string[])
        n226 = Less?(x=w486, y=i16 48) -> (x < y?=w501:bool)
        n227 = Array Subset(array=w476, index=w483, length=w481) -> (→"Data #":dbl[])
        n228 = call "GlobalIOData7.vi"("Function select"="Read All") -> ("Array"=w484:cluster{"Time":u32, "Value":sgl}[])  [unwired: 4 in, 1 out]
        n229 = Array Subset(array=w496, index=w493, length=24) -> (→"Array 2":string[])
        n230 = case shown="False" w501 {
          tunnel: w468 -> [w628 w675]
          tunnel: w450 -> [_ _]
          tunnel: "Page" -> [w625 w672]
          tunnel: w477 -> [w629 w665]
          tunnel: w450 -> [w627 w674]
          tunnel: w476 -> [w624 w673]
          tunnel: w475 -> [w626 w671]
          tunnel: w474 -> [w623 w670]
          tunnel: [w619 w669] -> w473
          tunnel: [w620 w668] -> w472
          tunnel: w471 -> [w622 w667]
          tunnel: [w621 w666] -> w470
          tunnel: w463 -> [_ w663]
          tunnel: w462 -> [_ w664]
          frame False {
            n231 = case shown="True" w628 {
              tunnel: w627 -> [_ w641]
              tunnel: w624 -> [_ w651]
              tunnel: w625 -> [_ w638]
              tunnel: w626 -> [w633 w650]
              tunnel: w623 -> [w632 w649]
              tunnel: [w632 w648] -> w620
              tunnel: [w633 w647] -> w619
              tunnel: w622 -> [w631 w646]
              tunnel: [w631 w645] -> w621
              tunnel: w629 -> [w630 w636]
              tunnel: [w630 w635] -> _
              frame False {
                # "The outer case structure being FALSE  indicates that the maximum of 48 data channels\nhas been reached"
                # "TRUE: Something has been eitehr selected or deselected \nFALSE: do nothing"
              }
              frame True {
                w634 = FALSE ("new element/subarray")
                n232 = Search 1D Array(1D array=w641, element=TRUE, start index (0)=0) -> (index of element=w643:i32)
                n233 = Multiply(x=24.0, y=w638) -> (x*y=w639:dbl)
                n234 = Add(x=w643, y=w639) -> (x+y=w637:dbl)
                n235 = Replace Array Subset(array=w636, new element=w634, index=w637) -> (w635:bool[])
                n236 = case shown="False" w634 {
                  tunnel: w651 -> [_ _]
                  tunnel: w650 -> [w658 w662]
                  tunnel: w649 -> [w657 w661]
                  tunnel: [w653 w661] -> w648
                  tunnel: [w654 w662] -> w647
                  tunnel: w646 -> [w656 w660]
                  tunnel: [w652 w660] -> w645
                  tunnel: w637 -> [w659 _]
                  frame False {
                    n237 = Search 1D Array(1D array=w658, element=w659) -> (index of element=w655:i32)  [unwired: 1 in]
                    n238 = Delete From Array(array=w658, index=w655) -> (array with subset deleted=w654:dbl[])  [unwired: 1 in, 1 out]
                    n239 = Delete From Array(array=w657, index=w655) -> (array with subset deleted=w653:dbl[])  [unwired: 1 in, 1 out]
                    n240 = Delete From Array(array=w656, index=w655) -> (array with subset deleted=w652:enum32{"Slow", "Medium", "Fast"}[])  [unwired: 1 in, 1 out]
                  }
                  frame True {
                    # "True: do nothing (array is full)\nFalse: remove from data array"
                  }
                }
                n241 = global write "GlobalDataSelectArray.vi" "Data Select Array"(w635) -> ()
              }
            }
          }
          frame True {
            n242 = case shown="False" w675 {
              tunnel: w674 -> [_ w690]
              tunnel: w673 -> [_ w700]
              tunnel: w672 -> [_ w687]
              tunnel: w671 -> [w679 w699]
              tunnel: w670 -> [w678 w698]
              tunnel: [w678 w697] -> w668
              tunnel: [w679 w696] -> w669
              tunnel: w667 -> [w677 w695]
              tunnel: [w677 w694] -> w666
              tunnel: w665 -> [w676 w684]
              tunnel: [w676 w682] -> _
              tunnel: w664 -> [_ w681]
              tunnel: w663 -> [_ w680]
              frame False {
                # "The outer case structure being TRUE  indicates that less than 48 data channels\nhave been selected"
                # "TRUE: Something has been either selected or deselected \nFALSE: do nothing"
              }
              frame True {
                n243 = Search 1D Array(1D array=w690, element=TRUE, start index (0)=0) -> (index of element=w692:i32)
                n244 = Multiply(x=24.0, y=w687) -> (x*y=w688:dbl)
                n245 = Add(x=w692, y=w688) -> (x+y=w686:dbl)
                n246 = Index Array(array=w684, index=w686) -> (element=w685:bool)
                n247 = Not(x=w685) -> (.not. x?=w683:bool)
                n248 = Replace Array Subset(array=w684, new element=w683, index=w686) -> (w682:bool[])
                n249 = case shown="True" w683 {
                  tunnel: w700 -> [_ w727]
                  tunnel: w699 -> [w716 w726]
                  tunnel: w698 -> [w715 w724]
                  tunnel: [w712 w723] -> w697
                  tunnel: [w713 w722] -> w696
                  tunnel: w695 -> [w714 w721]
                  tunnel: [w711 w720] -> w694
                  tunnel: w686 -> [w717 w719]
                  tunnel: w681 -> [w710 _]
                  tunnel: w680 -> [w709 _]
                  frame False {
                    w706 = 24 ("index")
                    n250 = Search 1D Array(1D array=w716, element=w717) -> (index of element=w708:i32)  [unwired: 1 in]
                    n251 = Delete From Array(array=w709, index=w708) -> (array with subset deleted=w705:bool[])  [unwired: 1 in, 1 out]
                    n252 = Delete From Array(array=w710, index=w708) -> (array with subset deleted=w707:bool[])  [unwired: 1 in, 1 out]
                    n253 = Delete From Array(array=w716, index=w708) -> (array with subset deleted=w713:dbl[])  [unwired: 1 in, 1 out]
                    n254 = Delete From Array(array=w715, index=w708) -> (array with subset deleted=w712:dbl[])  [unwired: 1 in, 1 out]
                    n255 = Delete From Array(array=w714, index=w708) -> (array with subset deleted=w711:enum32{"Slow", "Medium", "Fast"}[])  [unwired: 1 in, 1 out]
                    n256 = Split 1D Array(array=w705, index=w706) -> (first subarray=w702:bool[], second subarray=w701:bool[])
                    n257 = Split 1D Array(array=w707, index=w706) -> (first subarray=w704:bool[], second subarray=w703:bool[])
                    n258 = local write "One1"(w704) -> ()
                    n259 = local write "Two1"(w702) -> ()
                    n260 = local write "One2"(w703) -> ()
                    n261 = local write "Two2"(w701) -> ()
                  }
                  frame True {
                    # "True: add to data array\nFalse: remove from data array"
                    n262 = Index Array(array=w727, index=w719) -> (element=w725:dbl)
                    n263 = Build Array (concatenate)(w724, w725) -> (w723:dbl[])
                    n264 = Build Array (concatenate)(w726, w719) -> (w722:dbl[])
                    n265 = Build Array (concatenate)(w721, enum32{"Slow", "Medium", "Fast"}."Slow" ("Radio Buttons 2")) -> (w720:enum32{"Slow", "Medium", "Fast"}[])
                  }
                }
                n266 = global write "GlobalDataSelectArray.vi" "Data Select Array"(w682) -> ()
              }
            }
          }
        }
        n267 = for {
          tunnel: w476 -> [w609] mode=indexing
          tunnel: w484 -> [w610]
          tunnel: [w607] -> w480 mode=indexing
          # "Read in Values"
          n268 = Index Array(array=w610, index=w609) -> (element=w608:cluster{"Time":u32, "Value":sgl})
          n269 = Unbundle(w608) -> ("Value"=w607:sgl)  [unwired: 1 out]
        }
        n270 = Increment(x="Page") -> (x+1=w489:dbl)
        n271 = Multiply(x=w489, y=w490) -> (x*y=w482:dbl)
        n272 = Add(x=24.0 ("y"), y=w494) -> (x+y=w505:dbl)
        n273 = Array Subset(array=w476, index=w482, length=w490) -> (→"Data # 2":dbl[])
        n274 = Array Subset(array=w477, index=w494, length=24) -> (→"Indicator":bool[])
        n275 = Array Subset(array=w480, index=w482, length=w481) -> (→"Value 2":sgl[])
        n276 = Array Subset(array=w477, index=w505, length=24) -> (→"Indicator 2":bool[])
        n277 = Array Subset(array=w480, index=w483, length=w481) -> (→"Value 1":sgl[])
        n278 = case shown="False" FALSE {
          frame False {
            # "NOT FUNCTIONING YET!!\n\n\nTrue: Load saved data configuration\nfalse: do nothing"
            # "Need to write to global data num\nneed to reinitialize plot data table"
          }
          frame True {
            (unwired) enum16{"read/write", "read-only", "write-only"}."read-only" ("access (0:read/write)")
            w555 = enum32{"Slow", "Medium", "Fast"}[] [enum."Slow", enum."Slow", enum."Slow", enum."Slow", enum."Slow", enum."Slow", enum."Slow", enum."Slow", enum."Slow", enum."Slow", enum."Slow", enum."Slow", enum."Slow", enum."Slow", enum."Slow", enum."Slow", enum."Slow", enum."Slow", enum."Slow", enum."Slow", enum."Slow", enum."Slow", enum."Slow", enum."Slow"] items=["Slow", "Medium", "Fast"] ("Speed Sel 2")
            n279 = global read "GlobalDataSelectArray.vi" "Data Select Array"() -> (w540:bool[])
            n280 = Array Size(array=w540) -> (size(s)=w539:i32)
            n281 = Open/Create/Replace File(prompt="Please Select Data Channel File", operation (0:open)=T8."open") -> (refnum out=w543:refnum<file>)  [unwired: 4 in, 2 out]
            n282 = Read from Text File(file (use dialog)=w543) -> (refnum out=w547:refnum<file>, text=w545:string)  [unwired: 3 in, 2 out]
            n283 = Read from Text File(file (use dialog)=w547) -> (refnum out=w551:refnum<file>, text=w549:string, error out=w552:errorcluster)  [unwired: 3 in, 1 out]
            n284 = Close File(refnum=w551, error in=w552) -> ()  [unwired: 2 out]
            n285 = Initialize Array(FALSE, w539) -> (w537:bool[])
            n286 = Spreadsheet String To Array(format string="%d", spreadsheet string=w549, array type (2D Dbl)=w555) -> (array=w554:enum32{"Slow", "Medium", "Fast"}[])  [unwired: 1 in]
            n287 = Spreadsheet String To Array(format string="%d", spreadsheet string=w545, array type (2D Dbl)=sgl[] []) -> (array=w541:sgl[])  [unwired: 1 in]
            n288 = for {
              tunnel: w541 -> [w560] mode=indexing
              shift-right: [w558] -> w536
              shift-left: w537 -> [w561]
              n289 = Replace Array Subset(array=w561, new element=TRUE, index=w560) -> (w558:bool[])
            }
            n290 = global write "GlobalDisplayIndex.vi" "display address"(w541) -> ()
            n291 = Split 1D Array(array=w554, index=24) -> (first subarray=w556:enum32{"Slow", "Medium", "Fast"}[], second subarray=w557:enum32{"Slow", "Medium", "Fast"}[])
            n292 = local write "Speed Sel 2"(w557) -> ()
            n293 = local write "Speed Sel"(w556) -> ()
            n294 = global write "GlobalDataSelectArray.vi" "Data Select Array"(w536) -> ()
          }
        }
        n295 = global write "GlobalDisplayIndex.vi" "display address"(w473) -> ()
        n296 = global write "GlobalDisplayIndex.vi" "display canID"(w472) -> ()
        n297 = Split 1D Array(array=w470, index=24) -> (first subarray=w461:enum32{"Slow", "Medium", "Fast"}[], second subarray=w460:enum32{"Slow", "Medium", "Fast"}[])
        n298 = local write "Speed Sel 2"(w460) -> ()
        n299 = local write "Speed Sel"(w461) -> ()
        n300 = case shown="True" "Search \nButton" {
          frame False {
            # "True: Initialize search and return all search hits\nFalse: do nothing"
          }
          frame True {
            n301 = call "GlobalDataAddress.vi"("Function select"="Read All") -> ("Data ID Out"=w588:dbl[], "Data Names Out"=w590:string[])  [unwired: 3 in, 2 out]
            n302 = Initialize Array(T9 {"Numeric"=0.0, "String"="", "ignore case? (F)"=FALSE} ("cluster")) -> (w587:T12)  [unwired: 1 in]
            n303 = for {
              tunnel: w590 -> [w597] mode=indexing
              tunnel: w588 -> [w595] mode=indexing
              tunnel: "Search" -> [w599]
              shift-right: [w593] -> w586
              shift-left: w587 -> [w592]
              # "Search each Name for given string"
              n304 = Search and Replace String(case sensitive?=TRUE ("ignore case? (F)"), input string=w597, search string=w599) -> (number of replacements=w598:i32)  [unwired: 5 in, 3 out]
              n305 = Greater Than 0?(x=w598) -> (x > 0?=w596:bool)
              n306 = case shown="True" w596 {
                tunnel: w597 -> [_ w605]
                tunnel: w595 -> [_ w606]
                tunnel: [w600 w603] -> w593
                tunnel: w592 -> [w600 w602]
                frame False {
                }
                frame True {
                  n307 = Bundle("Numeric"=w606, "String"=w605, "ignore case? (F)"=FALSE) -> (w604:T9)  [unwired: 1 in]
                  n308 = Build Array (concatenate)(w602, w604) -> (w603:T12)
                }
              }
            }
            "Results" <- w586
            n309 = Array Size(array=w586) -> (size(s)=→"# of Results":i32)
          }
        }
        n310 = case shown="True" "save data" {
          frame False {
            # "NOT FUNCTIONING YET!!\n\n\nTrue: save data configuration\nfalse: do nothing"
          }
          frame True {
            w573 = "DataChannels.txt" ("Default file name")
            # "Generate time stamp"
            n311 = local read "Speed Sel"() -> (w582:enum32{"Slow", "Medium", "Fast"}[])
            n312 = local read "Speed Sel 2"() -> (w581:enum32{"Slow", "Medium", "Fast"}[])
            n313 = global read "GlobalDisplayIndex.vi" "display address"() -> (w578:dbl[])
            n314 = String Length(string=w573) -> (length=w571:i32)
            n315 = Format Date/Time String(time format string (%c)="-%Y%m%d-%H%M%S") -> (date/time string=w577:string)  [unwired: 2 in]
            n316 = Build Array (concatenate)(w582, w581) -> (w579:enum32{"Slow", "Medium", "Fast"}[])
            n317 = Subtract(x=w571, y=4) -> (x-y=w575:i32)
            n318 = Replace Substring(2:0, 3:w575, 4:w577, 5:w573) -> (1:w572:string)  [unwired: 1 out]
            n319 = Array To Spreadsheet String(array=w578, 3:"%d") -> (spreadsheet string=w563:string)  [unwired: 1 in]
            n320 = Array To Spreadsheet String(array=w579, 3:"%d") -> (spreadsheet string=w583:string)  [unwired: 1 in]
            n321 = File Dialog(9:w572) -> (0:w570:errorcluster, 3:w568:path)  [unwired: 6 in, 2 out]
            n322 = Unbundle(w570) -> ()  [unwired: 3 out]
            n323 = Open/Create/Replace File(file path (use dialog)=w568, operation (0:open)=T8."create") -> (refnum out=w566:refnum<file>)  [unwired: 4 in, 2 out]
            n324 = Write to Text File(file (use dialog)=w566, text=w563) -> (refnum out=w565:refnum<file>)  [unwired: 2 in, 2 out]
            n325 = Write to Text File(file (use dialog)=w565, text=w583) -> (refnum out=w564:refnum<file>)  [unwired: 2 in, 2 out]
            n326 = Close File(refnum=w564) -> ()  [unwired: 1 in, 2 out]
          }
        }
        n327 = case shown="True" w468 {
          tunnel: w472 -> [_ w612]
          frame False {
            # "True: Update plot table if a data channel\nhas been selected or deselected.\n\nFalse: do nothing"
          }
          frame True {
            n328 = flat-sequence {
              tunnel: w612 -> [w613]
              tunnel: [w613] -> w611
              tunnel: w611 -> [w615]
              frame #0 {
                n329 = call "GlobalPlotDataIDTable7.vi"("Function select"="Initialize") -> ()  [unwired: 3 in, 1 out]
              }
              frame #1 {
                n330 = for {
                  tunnel: w615 -> [w616] mode=indexing
                  i -> [w617]
                  n331 = call "GlobalPlotDataIDTable7.vi"("IO Data ID in"=w616, "Plot channel in"=w617, "Function select"="Write") -> ()  [unwired: 1 in, 1 out]
                }
              }
            }
          }
        }
        n332 = call "GlobalDataNum7.vi"("Data  Numbers In"=w472, "Function select"="Write All") -> ()  [unwired: 2 in, 2 out]
      }
      frame "Display Data" {
        # "Note: in order to set the speed you must assign a value of:\n\nVALUE = SPEEDVAL + CAN_ID# \n\nto the appropriate labview speed channel corresponding to the position\nof the data in the data table  \n\nSPEEDVAL is: \n                     0 for slow\n             65536 for medium\n           131072 for fast"
        # "Indexing the output here might be a problem\nwhen we're feeding into two different arrays..."
        # "Speed \"Translator\": Input a 48-element vector of data speed numbers. This function\nevaluates whether each number corresponds to a high, med, or low speed data \nvalue by checking what range it falls into. (Select range via \"range selectors\") Returns \na 48-element vector of color values, each either red, green, or yellow"
        n333 = global read "GlobalSpeedUpdateTime.vi" "Previous speed update time"() -> (w734:dbl)
        n334 = global read "GlobalDisplayIndex.vi" "display address"() -> (w737:dbl[])
        n335 = Tick Count (ms)() -> (millisecond timer value=w731:u32)
        n336 = Subtract(x=w731, y=w734) -> (x-y=w732:dbl)
        n337 = call "GlobalIOData7.vi"("Function select"="Read All") -> ("Array"=w735:cluster{"Time":u32, "Value":sgl}[])  [unwired: 4 in, 1 out]
        n338 = Greater?(x=w732, y=2000.0) -> (0:w730:bool)
        n339 = call "GlobalDataNum7.vi"("Function select"="Read All") -> ("Data Numbers Out"=w746:dbl[])  [unwired: 3 in, 1 out]
        n340 = Build Array (concatenate)("Speed Sel", "Speed Sel 2") -> (w752:enum32{"Slow", "Medium", "Fast"}[])
        n341 = for {
          N: 48 -> [_]
          tunnel: [w765] -> w751 mode=indexing
          tunnel: w752 -> [w754] mode=indexing
          tunnel: [w763] -> w745 mode=indexing
          tunnel: w746 -> [w758] mode=indexing
          tunnel: [w759] -> w741 mode=indexing
          tunnel: w737 -> [w755] mode=indexing
          tunnel: w735 -> [w762]
          tunnel: w731 -> [w757]
          tunnel: w730 -> [w756]
          tunnel: [w756] -> _
          i -> [w760]
          # "Reads and sets the data speeds based on what range\nthe values fall into."
          n342 = case shown="True" w756 {
            tunnel: [w766 w792] -> w765
            tunnel: w760 -> [w768 w790]
            tunnel: w758 -> [_ w786]
            tunnel: w757 -> [_ w785]
            tunnel: w754 -> [_ w771]
            frame False {
              n343 = local read "Speed 3"() -> (w769:u32[])
              n344 = local read "Speed 2"() -> (w770:u32[])
              n345 = Build Array (concatenate)(w770, w769) -> (w767:u32[])
              n346 = Index Array(array=w767, index=w768) -> (element=w766:u32)
            }
            frame True {
              n347 = global read "GlobalLabVIEWStart.vi" "LabVIEW Speed Channels"() -> (w791:dbl[])
              n348 = global write "GlobalSpeedUpdateTime.vi" "Previous speed update time"(w785) -> ()
              n349 = case shown="\"Fast\"" w771 {
                tunnel: [0 65536 131072] -> w787
                frame "Slow", Default {
                }
                frame "Medium" {
                }
                frame "Fast" {
                }
              }
              n350 = Index Array(array=w791, index=w790) -> (element=w783:dbl)
              n351 = Add(x=w787, y=w786) -> (x+y=w788:dbl)
              n352 = call "GlobalTransmitBuffer7.vi"("Data_ID # in"=w783, "Value in"=w788, "Function select"="Write") -> ()  [unwired: 3 out]
              n353 = call "GlobalIOData7.vi"("Function select"="Read One", "IO Data ID"=w783) -> ("IO data out"=w782:cluster{"Time":u32, "Value":sgl})  [unwired: 3 in, 1 out]
              n354 = Unbundle(w782) -> ("Value"=w781:sgl)  [unwired: 1 out]
              n355 = Less?(x=w781, y=sgl 5000.0) -> (x < y?=w778:bool)
              n356 = Less?(x=w781, y=sgl 70000.0) -> (x < y?=w777:bool)
              n357 = Select(t=1, s=w778, f=2) -> (s? t:f=w776:i32)
              n358 = Select(t=w776, s=w777, f=3) -> (s? t:f=w775:i32)
              n359 = case shown="2" w775 {
                tunnel: [w796 w800 w804] -> w792
                frame 1, Default {
                  # "Slow\n(red)"
                  n360 = call <vilib>:"RGB to Color.vi"("B"=u8 0, "G"=u8 0, "R"=u8 255) -> ("Color"=w796:u32)
                }
                frame 2 {
                  # "Medium\n(yellow)"
                  n361 = call <vilib>:"RGB to Color.vi"("B"=u8 0, "G"=u8 255, "R"=u8 255) -> ("Color"=w800:u32)
                }
                frame 3 {
                  # "Fast\n(green)"
                  n362 = call <vilib>:"RGB to Color.vi"("B"=u8 0, "G"=u8 255, "R"=u8 0) -> ("Color"=w804:u32)
                }
              }
            }
          }
          n363 = Index Array(array=w762, index=w758) -> (element=w761:cluster{"Time":u32, "Value":sgl})
          n364 = Unbundle(w761) -> ("Value"=w759:sgl)  [unwired: 1 out]
          n365 = call "GlobalDataAddress.vi"("Element index"=w755, "Function select"="Read One") -> ("Data name"=w763:string)  [unwired: 2 in, 3 out]
        }
        n366 = Split 1D Array(array=w751, index=24) -> (first subarray=→"Speed 2":u32[], second subarray=→"Speed 3":u32[])
        n367 = Split 1D Array(array=w745, index=24) -> (first subarray=→"Data Names 1":string[], second subarray=→"Data Names 2":string[])
        n368 = Split 1D Array(array=w741, index=24) -> (first subarray=→"Data Value 1":sgl[], second subarray=→"Data Value 2":sgl[])
      }
      frame "SUGGESTIONS" {
      }
      frame "Errors" {
      }
    }
    n369 = global read "GlobalBatteryVoltageID.vi" "Batt Voltage ID"() -> (w65:dbl)
    n370 = flat-sequence {
      tunnel: [w134] -> w74
      tunnel: w74 -> [w140]
      frame #0 {
        n371 = call "GlobalIOData7.vi"("Function select"="Read One", "IO Data ID"=u32 0) -> ("IO data out"=w130:cluster{"Time":u32, "Value":sgl})  [unwired: 3 in, 1 out]
        n372 = Unbundle(w130) -> ("Value"=w129:sgl)  [unwired: 1 out]
        n373 = call "GlobalMCUmS7.vi"("mS In"=w129, "Function select"="Write") -> ()  [unwired: 2 out]
      }
      frame #1 {
        # "This runs the timer display and checks if the robot is turned off"
        n374 = global read "GlobalRobotOffCheck.vi" "Previous Timestamp"() -> (w136:dbl)
        n375 = call "GlobalMCUmS7.vi"("Function select"="Read One") -> ("mS Out"=w133:u32)  [unwired: 1 in, 1 out]
        "MCU Elapsed mS 2" <- w133
        n376 = Divide(x=w133, y=u32 1000) -> (x/y=w134:dbl)
        "MCU Elapsed mS" <- w134
        n377 = Less?(x=w134, y=w136) -> (x < y?=w137:bool)
        n378 = case shown="True" w137 {
          frame False {
          }
          frame True {
            n379 = local write "Collect Data"(FALSE ("Collect Data")) -> ()
          }
        }
      }
      frame #2 {
        n380 = global write "GlobalRobotOffCheck.vi" "Previous Timestamp"(w140) -> ()
      }
    }
    n381 = case shown="True" "Collect Data" {
      selector: "Collect Data" -> [w808 w813]
      frame False {
        # "True: data collection on\nFalse: data collection off"
        n382 = call "GlobSave2File7.vi"("Function select"="Clear") -> ()  [unwired: 1 out]
        n383 = local write "Boolean"(w808) -> ()
      }
      frame True {
        # "Creates new file each time turned on"
        # "Turns data collection on/off"
        n384 = flat-sequence {
          tunnel: w813 -> [w815]
          tunnel: [w815] -> w812
          tunnel: [w814] -> w810
          tunnel: w812 -> [w818]
          tunnel: [w818] -> w811
          tunnel: w810 -> [w817]
          tunnel: w811 -> [w832]
          frame #0 {
            n385 = local read "Boolean"() -> (w814:bool)
            n386 = call "GlobSave2File7.vi"("Function select"="Set") -> ()  [unwired: 1 out]
          }
          frame #1 {
            n387 = Not Equal?(x=w818, y=w817) -> (x != y?=w819:bool)
            n388 = case shown="True" w819 {
              frame False {
              }
              frame True {
                n389 = flat-sequence {
                  frame #0 {
                    # "Generate time stamp for file"
                    n390 = global read "GlobalDataPath7.vi" "Data File Path"() -> (w820:path)
                    n391 = Path To String(path=w820) -> (string=w830:string)
                    n392 = String Length(string=w830) -> (length=w823:i32)
                    n393 = Subtract(x=w823, y=4) -> (x-y=w825:i32)
                    n394 = Format Date/Time String(time format string (%c)="-%Y%m%d-%H%M%S") -> (date/time string=w829:string)  [unwired: 2 in]
                    n395 = Replace Substring(2:0, 3:w825, 4:w829, 5:w830) -> (1:w827:string)  [unwired: 1 out]
                    n396 = String To Path(string=w827) -> (path=w831:path)
                    n397 = Open/Create/Replace File(file path (use dialog)=w831, operation (0:open)=5) -> (refnum out=w822:refnum<file>)  [unwired: 4 in, 2 out]
                    n398 = global write "GlobalDataFileRefnum7.vi" "Data File Refnum"(w822) -> ()
                  }
                  frame #1 {
                    n399 = call "AppendParamNamesNumbers.vi"() -> ()  [unwired: 12 in]
                  }
                }
              }
            }
          }
          frame #2 {
            "Boolean" <- w832
          }
        }
      }
    }
    n400 = call "GlobalIOData7.vi"("Function select"="Read One", "IO Data ID"=w65) -> ("IO data out"=w66:cluster{"Time":u32, "Value":sgl})  [unwired: 3 in, 1 out]
    n401 = Unbundle(w66) -> ("Value"=→"BATTERY VOLTAGE":sgl)  [unwired: 1 out]
    n402 = call "GlobalDataNum7.vi"("Function select"="Read All") -> ("Data Numbers Out"=w77:dbl[])  [unwired: 3 in, 1 out]
    n403 = Array Subset(array=w77, index=0, length=24) -> (→"Channel # 1":dbl[])
    n404 = Array Subset(array=w77, index=24, length=24) -> (→"Channel # 2":dbl[])
    n405 = Build Array (concatenate)("Two1", "Two2") -> (w79:bool[])
    n406 = Build Array (concatenate)("One1", "One2") -> (w78:bool[])
    n407 = case shown="True" "Graph\non" {
      tunnel: w77 -> [_ w146]
      tunnel: w79 -> [_ w147]
      frame False {
        # "This case structure deals with all the graphing for graph 2"
      }
      frame True {
        # "Output of Names"
        # "Output of Values"
        # "GRAPH 2"
        # "Local Index Selector"
        n408 = Initialize Array(0.0 ("element")) -> (w141:dbl[])  [unwired: 1 in]
        n409 = Initialize Array(0 ("index of element")) -> (w144:i32[])  [unwired: 1 in]
        n410 = while {
          tunnel: w147 -> [w175]
          shift-right: [w160] -> _
          shift-left: 0 ("index of element") -> [w162]
          tunnel: w146 -> [w169]
          shift-right: [w165] -> w150
          shift-left: w141 -> [w170]
          shift-right: [w157] -> w149
          shift-left: w141 -> [w158]
          shift-right: [w156] -> w148
          shift-left: w144 -> [w155]
          stop <- w163 stop-if-true
          n411 = global read "GlobalDisplayIndex.vi" "display address"() -> (w159:dbl[])
          n412 = Search 1D Array(1D array=w175, element=TRUE, start index (0)=w162) -> (index of element=w161:i32)
          n413 = Not Equal?(x=w161, y=-1.0) -> (x != y?=w171:bool)
          n414 = case shown="True" w171 {
            tunnel: w161 -> [_ w183]
            tunnel: w170 -> [w178 w188]
            tunnel: w169 -> [_ w189]
            tunnel: [w178 w187] -> w165
            tunnel: w159 -> [_ w180]
            tunnel: w158 -> [w177 w185]
            tunnel: [w177 w184] -> w157
            tunnel: [w176 w182] -> w156
            tunnel: w155 -> [w176 w181]
            frame False {
            }
            frame True {
              n415 = Index Array(array=w189, index=w183) -> (element=w186:dbl)
              n416 = Index Array(array=w180, index=w183) -> (element=w179:dbl)
              n417 = Build Array (concatenate)(w181, w183) -> (w182:i32[])
              n418 = Build Array (concatenate)(w188, w186) -> (w187:dbl[])
              n419 = Build Array (concatenate)(w185, w179) -> (w184:dbl[])
            }
          }
          n420 = Array Size(array=w165) -> (size(s)=w166:i32)
          n421 = Increment(x=w161) -> (x+1=w160:i32)
          n422 = Equal?(x=w161, y=-1.0) -> (x = y?=w168:bool)
          n423 = Equal?(x=4.0, y=w166) -> (x = y?=w164:bool)
          n424 = Or(x=w168, y=w164) -> (x .or. y?=w163:bool)
        }
        n425 = call "GlobalDataAddress.vi"("Function select"="Read All") -> ("Data Names Out"=w154:string[])  [unwired: 3 in, 3 out]
        n426 = for {
          tunnel: w154 -> [w195]
          tunnel: [w194] -> w152 mode=indexing
          tunnel: [w192] -> w153 mode=indexing
          tunnel: w150 -> [_] mode=indexing
          tunnel: w149 -> [w191] mode=indexing
          tunnel: w148 -> [w190] mode=indexing
          n427 = Index Array(array=w195, index=w191) -> (element=w194:string)
          n428 = call "GlobalPlotData7.vi"("Function select"="Read", "Data channel #"=w190) -> ("Single data plot cluster"=w192:cluster{"Array":u32[], "Array 2":sgl[]})  [unwired: 3 in]
        }
        "Graph Two" <- w153
        "graph2labels" <- w152
      }
    }
    n429 = case shown="True" "Graph\non" {
      tunnel: w77 -> [_ w206]
      tunnel: w78 -> [_ w205]
      frame False {
        # "This case structure deals with all the graphing for graph 1"
      }
      frame True {
        # "GRAPH 1"
        # "Output of Names"
        # "Output of Values"
        # "Local Index Selector"
        # "Global Index Selector"
        n430 = Initialize Array(0 ("index of element")) -> (w198:i32[])  [unwired: 1 in]
        n431 = Initialize Array(0.0 ("element")) -> (w201:dbl[])  [unwired: 1 in]
        n432 = while {
          tunnel: w205 -> [w230]
          shift-right: [w215] -> _
          shift-left: 0 ("index of element") -> [w217]
          tunnel: w206 -> [w224]
          shift-right: [w220] -> w207
          shift-left: w201 -> [w225]
          shift-right: [w212] -> w200
          shift-left: w201 -> [w213]
          shift-right: [w211] -> w196
          shift-left: w198 -> [w210]
          stop <- w218 stop-if-true
          n433 = global read "GlobalDisplayIndex.vi" "display address"() -> (w214:dbl[])
          n434 = Search 1D Array(1D array=w230, element=TRUE, start index (0)=w217) -> (index of element=w216:i32)
          n435 = Not Equal?(x=w216, y=-1.0) -> (x != y?=w226:bool)
          n436 = case shown="True" w226 {
            tunnel: w216 -> [_ w238]
            tunnel: w225 -> [w233 w243]
            tunnel: w224 -> [_ w244]
            tunnel: [w233 w242] -> w220
            tunnel: w214 -> [_ w235]
            tunnel: w213 -> [w232 w240]
            tunnel: [w232 w239] -> w212
            tunnel: [w231 w237] -> w211
            tunnel: w210 -> [w231 w236]
            frame False {
            }
            frame True {
              n437 = Index Array(array=w235, index=w238) -> (element=w234:dbl)
              n438 = Index Array(array=w244, index=w238) -> (element=w241:dbl)
              n439 = Build Array (concatenate)(w236, w238) -> (w237:i32[])
              n440 = Build Array (concatenate)(w240, w234) -> (w239:dbl[])
              n441 = Build Array (concatenate)(w243, w241) -> (w242:dbl[])
            }
          }
          n442 = Array Size(array=w220) -> (size(s)=w221:i32)
          n443 = Increment(x=w216) -> (x+1=w215:i32)
          n444 = Equal?(x=w216, y=-1.0) -> (x = y?=w223:bool)
          n445 = Equal?(x=4.0, y=w221) -> (x = y?=w219:bool)
          n446 = Or(x=w223, y=w219) -> (x .or. y?=w218:bool)
        }
        n447 = call "GlobalDataAddress.vi"("Function select"="Read All") -> ("Data Names Out"=w209:string[])  [unwired: 3 in, 3 out]
        n448 = for {
          tunnel: w209 -> [w249]
          tunnel: w200 -> [w250] mode=indexing
          tunnel: [w248] -> w204 mode=indexing
          tunnel: [w246] -> w208 mode=indexing
          tunnel: w207 -> [_] mode=indexing
          tunnel: w196 -> [w245] mode=indexing
          n449 = Index Array(array=w249, index=w250) -> (element=w248:string)
          n450 = call "GlobalPlotData7.vi"("Function select"="Read", "Data channel #"=w245) -> ("Single data plot cluster"=w246:cluster{"Array":u32[], "Array 2":sgl[]})  [unwired: 3 in]
        }
        "Graph One" <- w208
        "graph1labels" <- w204
      }
    }
    n451 = global read "GlobalPlotUpdateTime.vi" "Prev Time"() -> (w71:dbl)
    n452 = Tick Count (ms)() -> (millisecond timer value=w72:u32)
    n453 = call "ErrorHandlerREADALL.vi"() -> ("Small Error Cluster Out"=w62:T7)  [unwired: 10 in, 1 out]
    n454 = case shown="False" "Clear Errors" {
      frame False {
        # "True: reset error variables\nFalse: do nothing"
      }
      frame True {
        n455 = global write "GlobalErrorCluster.vi" "Medium Error Cluster"(T7 [] ("Medium Error Cluster")) -> ()
        n456 = global write "GlobalErrorCluster.vi" "Cluster Timestamps"(dbl[] [] ("Cluster Timestamps")) -> ()
      }
    }
    n457 = call "ErrorHandlerUpdate.vi"("Small Input Cluster"=w62) -> ("Unsorted Timestamps"=w61:dbl[], "Full Error Cluster"=w60:T7)  [unwired: 9 in]
    n458 = call "GlobalStop7.vi"("Function select"="Read") -> ("stop"=w92:bool)
    n459 = Subtract(x=w72, y=w71) -> (x-y=w70:dbl)
    n460 = Greater?(x=w70, y=2000.0) -> (0:w68:bool)
    n461 = call "ErrorClusterSort2.vi"("Unsorted Timestamps"=w61, "Unsorted Errors"=w60) -> ("Sorted Timestamps"=w59:dbl[], "Sorted Errors"=w58:T7)  [unwired: 7 in]
    n462 = global write "GlobalErrorCluster.vi" "Cluster Timestamps"(w59) -> ()
    n463 = global write "GlobalErrorCluster.vi" "Medium Error Cluster"(w58) -> ()
    n464 = case shown="True" w68 {
      selector: w68 -> [w98 w110]
      frame False {
        # "True: cycle to next error message every 2 seconds\nFalse: keep displaying current error message"
        n465 = local write "error message"(w98) -> ()
      }
      frame True {
        n466 = Tick Count (ms)() -> (millisecond timer value=w99:u32)
        n467 = global read "GlobalErrorIndex.vi" "Err Index"() -> (w104:dbl)
        n468 = global read "GlobalErrorCluster.vi" "Medium Error Cluster"() -> (w107:T7)
        n469 = Array Size(array=w107) -> (size(s)=w105:i32)
        n470 = Decrement(x=w105) -> (x-1=w103:i32)
        n471 = global write "GlobalPlotUpdateTime.vi" "Prev Time"(w99) -> ()
        n472 = Greater?(x=w104, y=w103) -> (0:w102:bool)
        n473 = Select(t=0.0, s=w102, f=w104) -> (s? t:f=w100:dbl)
        n474 = Increment(x=w100) -> (x+1=w101:dbl)
        n475 = Array Subset(array=w107, index=w100, length=1) -> (w115:T7)
        n476 = call "ErrorHandlerLabel.vi"("Sorted Errors"=w115) -> ("Error Cluster Out"=w113:T13)  [unwired: 10 in]
        n477 = Index Array(array=w113, index=0) -> (element=w111:T14)
        n478 = Unbundle(w111) -> ("Error Name"=→"Error Name 1":string, "Board Name"=→"Board Name 1":string)  [unwired: 4 out]
        n479 = global write "GlobalErrorIndex.vi" "Err Index"(w101) -> ()
        "error message" <- w110
      }
    }
    n480 = call "ErrorHandlerLabel.vi"("Sorted Errors"=w58) -> ("Error Cluster Out"=w57:T13)  [unwired: 10 in]
    n481 = Wait Until Next ms Multiple(millisecond multiple=100) -> ()  [unwired: 1 out]
    n482 = case shown="False" "Pause Button" {
      tunnel: w57 -> [w116 _]
      frame False {
        n483 = for {
          tunnel: [w127] -> w121 mode=indexing
          tunnel: [w126] -> w120 mode=indexing
          tunnel: [w125] -> w119 mode=indexing
          tunnel: [w124] -> w118 mode=indexing
          tunnel: [w122] -> w117 mode=indexing
          tunnel: w116 -> [w123] mode=indexing
          n484 = Unbundle(w123) -> ("Frequency"=w127:dbl, "Description"=w126:string, "Error Name"=w125:string, "Board Name"=w124:string, "Timestamp"=w122:dbl)  [unwired: 1 out]
        }
        "Error Description" <- w120
        "Board" <- w118
        "Error Name" <- w119
        "Freq." <- w121
        "Time" <- w117
      }
      frame True {
        # "True: pause screen\nFalse: update fields"
      }
    }
    n485 = case shown="True" "stop" {
      frame False {
      }
      frame True {
        n486 = call "GlobalStop7.vi"("Function select"="Set") -> ()  [unwired: 1 out]
      }
    }
  }
